vi "PM_List_Window.vi"(4 "Array":string[](array[string])) -> (1 "Resource Name Out":string)   [LabVIEW 2021]
doc: "This VI is a Window with a list of USB devices.\nTo choose the device, select it from the list and click OK.\n\nInput:\n(1) Array - the devices name array.\n\nOutput:\n(1) Resource Name Out - the name of the selected device."
panel:
  in  "Select PM:":string(combo)
  in  "Cancel Button":bool
  in  "OK":bool
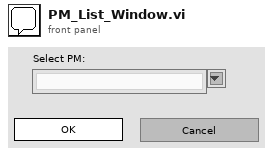
[diagram p1: front panel]
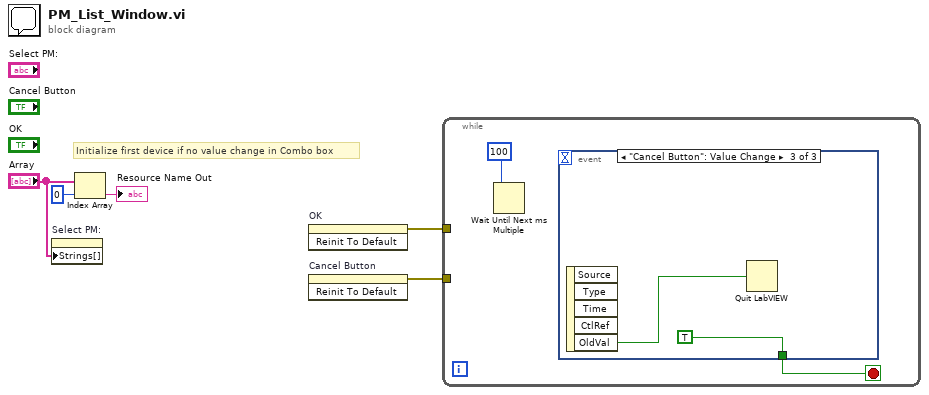
[diagram p0: block diagram]
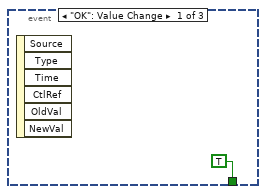
[diagram p2: hidden frame]
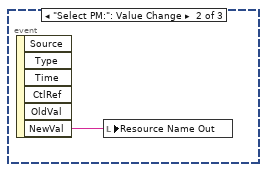
[diagram p3: hidden frame]
diagram:
  # "Initialize first device if no value change in Combo box"
  n1 = property on="Select PM:" class="CmbBox"("Strings[]"="Array") -> ()  [unwired: 2 in, 2 out]
  n2 = Index Array(array="Array", index=0) -> (element=→"Resource Name Out":string)
  n3 = invoke on="OK" class="Bool" method="Reinit To Default"() -> (error out=w5:errorcluster)  [unwired: 3 in, 2 out]
  n4 = invoke on="Cancel Button" class="Bool" method="Reinit To Default"() -> (error out=w4:errorcluster)  [unwired: 3 in, 2 out]
  n5 = while {
    tunnel: w5 -> [_]
    tunnel: w4 -> [_]
    stop <- w6 stop-if-true
    n6 = Wait Until Next ms Multiple(millisecond multiple=100) -> ()  [unwired: 1 out]
    n7 = event shown="[2] \"Cancel Button\": Value Change" {
      selector: _ -> [_ _ _]
      dyn-events: _ -> [_ _ _]
      timeout: _ -> [_ _ _]
      tunnel: [TRUE _ TRUE] -> w6
      event "OK": Value Change {
        n8 = event-data() -> ()  [unwired: 7 out]
      }
      event "Select PM:": Value Change {
        n9 = event-data() -> ("NewVal"=w9:string)  [unwired: 6 out]
        n10 = local write "Resource Name Out"(w9) -> ()
      }
      event "Cancel Button": Value Change {
        n11 = event-data() -> ("OldVal"=w10:bool)  [unwired: 5 out]
        n12 = Quit LabVIEW(quit? (T)=w10) -> ()
      }
    }
  }
